vi "Slice 1D Array (ENUM)__ogtk.vi"(5 "slice":string caption="subset (i:j)", 6 "array":enum16{"0", "1"}[](array[ring])) -> (1 "subarray (array[i:j])":enum16{"0", "1"}[](array[ring]))   [LabVIEW 2016]
doc: "Returns a subset from <B>array</B>. <B>subset</B> has the following syntax:\n\narray[subset] = subarray\n\nsubset is a range and is of the form \"i:j\" where i and j are integers\nif i is ommitted it is assumed to be zero. If j is ommitted it is assumed to be length(array)\nif i or j are negative numbers they are assumed to be refferenced from the end of the string.\nexamples:\n\nif array = [7,6,5,4,3,2,1]\n\nstring[2:] = [5,4,3,2,1]\nstring[:3] = [7,6,5]\nstring[-1] = [1]\nstring[4] = [3]\nstring[-4:-2] = [4,3]"
uses:
  <userlib>/_OpenG.lib/string/string.llb/Trim Whitespace (String)__ogtk.vi
panel:
  # "Slice 1D Array.vi\n\nReturns a subset from array\n\nPlease visit http://www.OpenG.org to learn about the\nOpen Source LabVIEW software movement.\n\nNOTICE -- YOU MUST LEAVE THIS NOTICE IN PLACE.  PER THE TERMS OF THE LICENSE BELOW, YOU MAY SUBLICENSE THIS SOFTWARE \nIN ANY WAY THAT DOES NOT CONFLICT WITH THIS LICENSE.\n\n### BSD License (http://www.opensource.org/licenses/bsd-license.php) Begin ###\n \nCopyright (c) 2002, Jim Kring <jim@jimkring.com>\nCopyright (c) 2002, Cal-Bay Systems, Inc. <info@calbay.com>\n\nAll rights reserved.\n\nRedistribution and use in source and binary forms, with or without modification, are permitted provided that the following conditions are met:\n\n    * Redistributions of source code must retain the above copyright notice, this list of conditions and the following disclaimer.\n    * Redistributions in binary form must reproduce the above copyright notice, this list of conditions and the following disclaimer in the \n       documentation and/or other materials provided with the distribution.\n    * Neither the name of SciWare, James Kring, Inc., nor the names of its contributors may be used to endorse or promote products derived \n       from this software without specific prior written permission.\n\nTHIS SOFTWARE IS PROVIDED BY THE COPYRIGHT HOLDERS AND CONTRIBUTORS \"AS IS\" AND ANY EXPRESS OR IMPLIED WARRANTIES, \nINCLUDING, BUT NOT LIMITED TO, THE IMPLIED WARRANTIES OF MERCHANTABILITY AND FITNESS FOR A PARTICULAR PURPOSE ARE \nDISCLAIMED. IN NO EVENT SHALL THE COPYRIGHT OWNER OR CONTRIBUTORS BE LIABLE FOR ANY DIRECT, INDIRECT, INCIDENTAL,\n SPECIAL, EXEMPLARY, OR CONSEQUENTIAL DAMAGES (INCLUDING, BUT NOT LIMITED TO, PROCUREMENT OF SUBSTITUTE GOODS OR \nSERVICES; LOSS OF USE, DATA, OR PROFITS; OR BUSINESS INTERRUPTION) HOWEVER CAUSED AND ON ANY THEORY OF LIABILITY, \nWHETHER IN CONTRACT, STRICT LIABILITY, OR TORT (INCLUDING NEGLIGENCE OR OTHERWISE) ARISING IN ANY WAY OUT OF THE USE \nOF THIS SOFTWARE, EVEN IF ADVISED OF THE POSSIBILITY OF SUCH DAMAGE.\n\n### BSD License End ###"
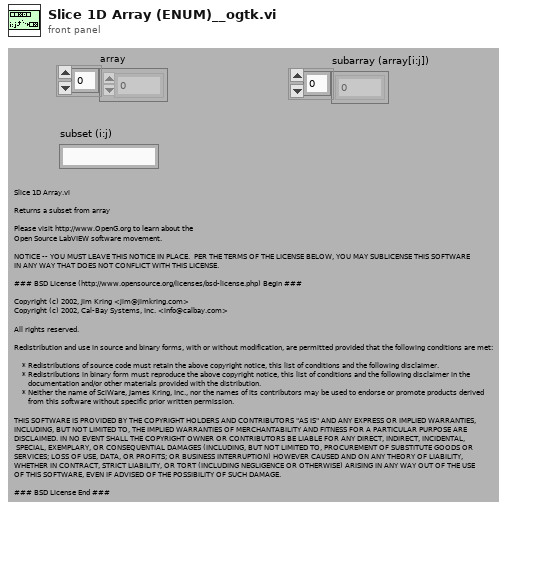
[diagram p1: front panel]
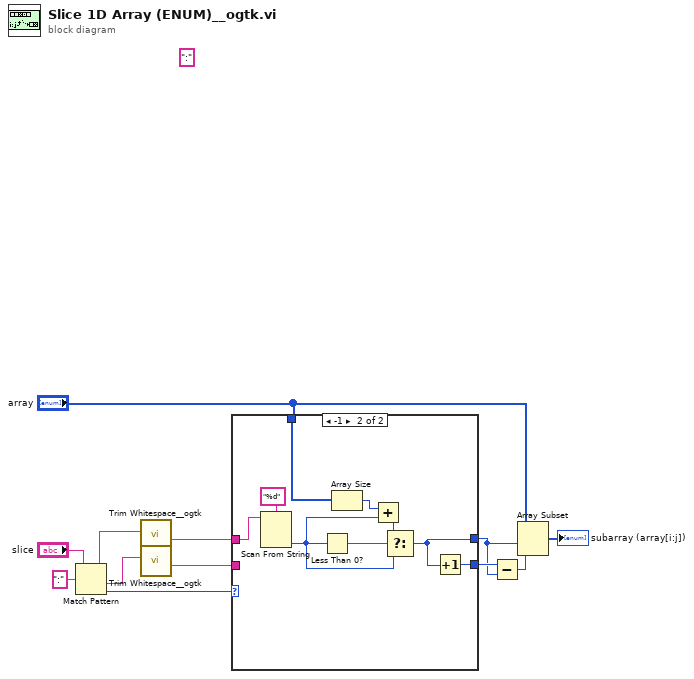
[diagram p0: block diagram]
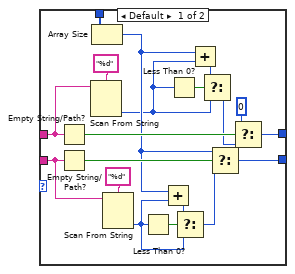
[diagram p2: hidden frame]
diagram:
  (unwired) ":"
  n1 = Match Pattern(string="slice", regular expression=":" ("search string/char (-)")) -> (before substring=w6:string, after substring=w4:string, offset past match=w7:i32)  [unwired: 1 in, 1 out]
  n2 = call-poly <userlib>:"Trim Whitespace__ogtk.vi"("String in"=w6) -> ("String out"=w5:string)  [unwired: 6 in]
  n3 = call-poly <userlib>:"Trim Whitespace__ogtk.vi"("String in"=w4) -> ("String out"=w3:string)  [unwired: 6 in]
  n4 = case shown="-1" w7 {
    tunnel: [w22 w33] -> w12
    tunnel: [w23 w32] -> w11
    tunnel: "array" -> [w28 w38]
    tunnel: w5 -> [w25 w39]
    tunnel: w3 -> [w29 _]
    frame Default {
      n5 = Empty String/Path?(string/path=w25) -> (empty?=w27:bool)
      n6 = Empty String/Path?(string/path=w29) -> (empty?=w31:bool)
      n7 = Scan From String(format string="%d" ("Format String"), input string=w25) -> (output 1=w14:i32)  [unwired: 3 in, 3 out]
      n8 = Array Size(array=w28) -> (size(s)=w16:i32)
      n9 = Scan From String(format string="%d" ("Format String"), input string=w29) -> (output 1=w19:i32)  [unwired: 3 in, 3 out]
      n10 = Less Than 0?(x=w19) -> (x < 0?=w21:bool)
      n11 = Add(x=w16, y=w19) -> (x+y=w20:i32)
      n12 = Less Than 0?(x=w14) -> (x < 0?=w17:bool)
      n13 = Select(t=w20, s=w21, f=w19) -> (s? t:f=w18:i32)
      n14 = Add(x=w16, y=w14) -> (x+y=w15:i32)
      n15 = Select(t=w15, s=w17, f=w14) -> (s? t:f=w13:i32)
      n16 = Select(t=w16, s=w31, f=w18) -> (s? t:f=w22:i32)
      n17 = Select(t=0 ("length"), s=w27, f=w13) -> (s? t:f=w23:i32)
    }
    frame -1 {
      n18 = Scan From String(format string="%d" ("Format String"), input string=w39) -> (output 1=w34:i32)  [unwired: 3 in, 3 out]
      n19 = Less Than 0?(x=w34) -> (x < 0?=w37:bool)
      n20 = Array Size(array=w38) -> (size(s)=w36:i32)
      n21 = Add(x=w36, y=w34) -> (x+y=w35:i32)
      n22 = Select(t=w35, s=w37, f=w34) -> (s? t:f=w32:i32)
      n23 = Increment(x=w32) -> (x+1=w33:i32)
    }
  }
  n24 = Subtract(x=w12, y=w11) -> (x-y=w2:i32)
  n25 = Array Subset(array="array", index=w11, length=w2) -> (→"subarray (array[i:j])":enum16{"0", "1"}[])
